vi "Enable.vi"(8 "output cluster":T1, 11 "Enum":T2=enum."Create Report") -> ()   [LabVIEW 2014]
uses:
  CMD UI enum.ctl
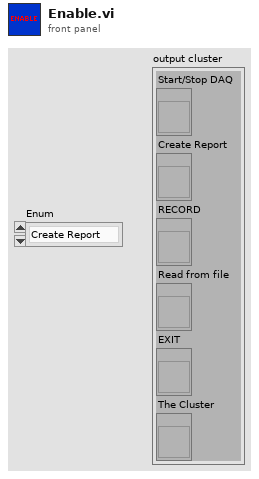
[diagram p1: front panel]
types:
  T1 = cluster{"Start/Stop DAQ":refnum<vi>, "Create Report":refnum<vi>, "RECORD":refnum<vi>, "Read from file":refnum<vi>, "EXIT":refnum<vi>, "The Cluster":refnum<vi>}
  T2 = typedef "CMD UI enum.ctl" = enum16{"Init all", "Update Patient Info", "Update Analyzed", "Create Report", "Analyze Data", "Start DAQ", "Start Read", "LOG Data", "Stop LOG Data", "Stop DAQ", "Stop Read", "EXIT"}
  T3 = enum8{"Enabled", "Disabled", "Disabled and Grayed Out"}
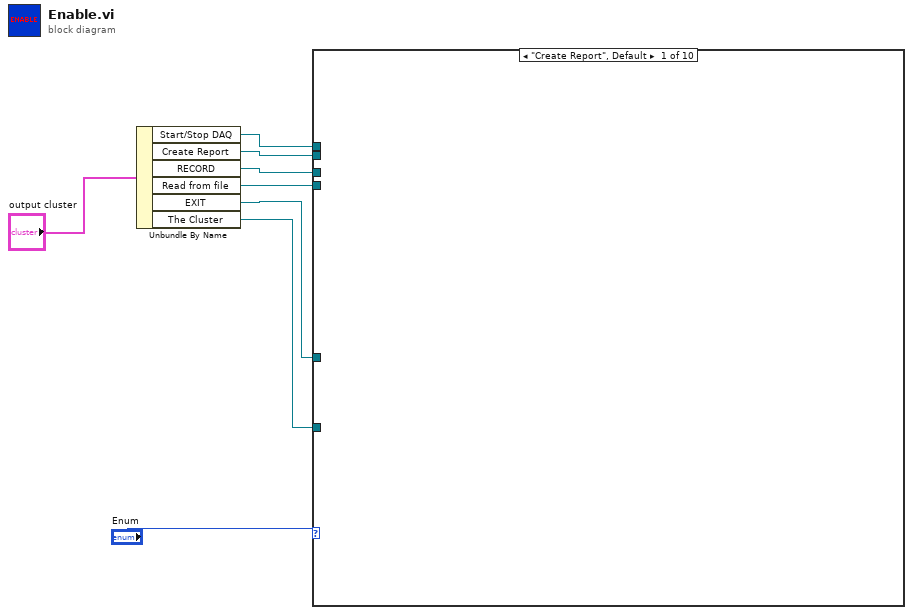
[diagram p0: block diagram]
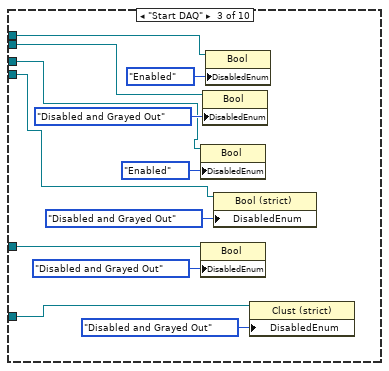
[diagram p3: hidden frame]
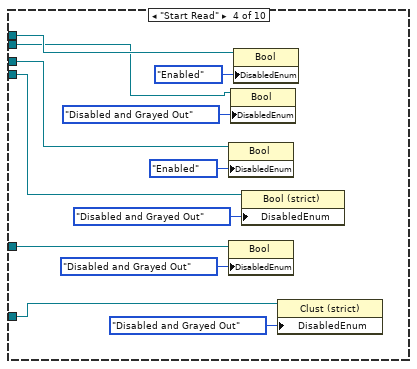
[diagram p4: hidden frame]
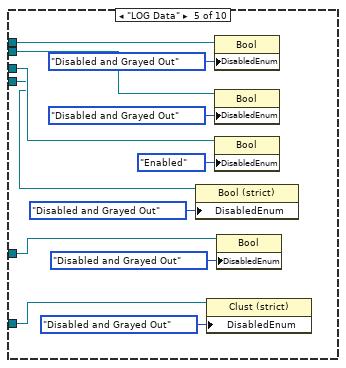
[diagram p5: hidden frame]
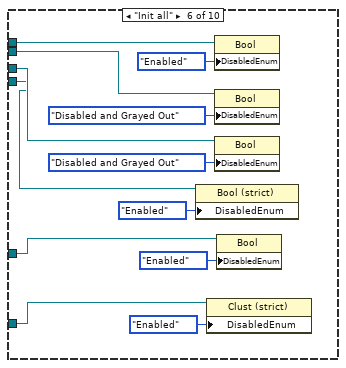
[diagram p6: hidden frame]
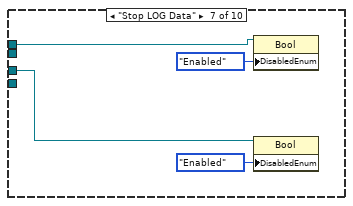
[diagram p7: hidden frame]
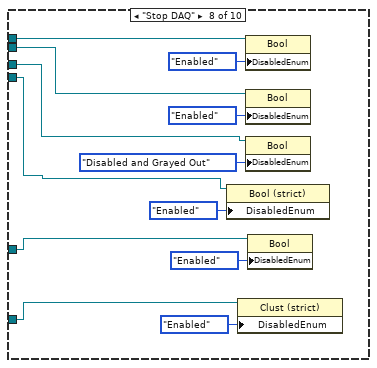
[diagram p8: hidden frame]
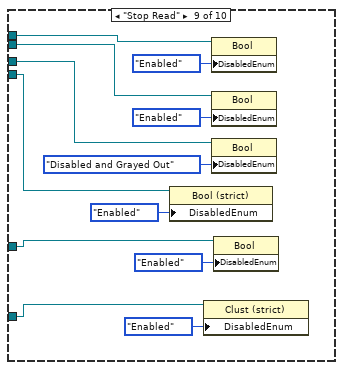
[diagram p9: hidden frame]
diagram:
  n1 = Unbundle By Name("output cluster") -> ("Start/Stop DAQ"=w7:refnum<vi>, "Create Report"=w6:refnum<vi>, "RECORD"=w5:refnum<vi>, "Read from file"=w3:refnum<vi>, "EXIT"=w2:refnum<vi>, "The Cluster"=w4:refnum<vi>)
  n2 = case shown="\"Create Report\", Default" "Enum" {
    tunnel: w7 -> [_ _ w15 w26 w44 w56 w58 w66 w78 _]
    tunnel: w6 -> [_ _ w14 w25 w43 w55 _ w65 w77 _]
    tunnel: w5 -> [_ _ w13 w24 w42 w54 w57 w64 w76 _]
    tunnel: w2 -> [_ _ w12 w22 w39 w51 _ w62 w74 _]
    tunnel: w4 -> [_ _ w10 w21 w40 w52 _ w61 w73 _]
    tunnel: w3 -> [_ _ w9 w23 w41 w53 _ w63 w75 _]
    frame "Create Report", Default {
    }
    frame "Analyze Data" {
    }
    frame "Start DAQ" {
      n3 = property on="Property Node" class="Bool"(reference=w13, "DisabledEnum"=T3."Enabled" ("Disabled")) -> ()  [unwired: 1 in, 2 out]
      n4 = property on="Property Node" class="Bool"(reference=w12, "DisabledEnum"=T3."Disabled and Grayed Out" ("Disabled")) -> ()  [unwired: 1 in, 2 out]
      n5 = property on="Property Node" class="Bool"(reference=w14, "DisabledEnum"=T3."Disabled and Grayed Out" ("Disabled")) -> ()  [unwired: 1 in, 2 out]
      n6 = property on="Property Node" class="Bool"(reference=w15, "DisabledEnum"=T3."Enabled" ("Disabled")) -> ()  [unwired: 1 in, 2 out]
      n7 = property on="Property Node" class="Bool (strict)"(reference=w9, "DisabledEnum"=T3."Disabled and Grayed Out" ("Disabled")) -> ()  [unwired: 1 in, 2 out]
      n8 = property on="Property Node" class="Clust (strict)"(reference=w10, "DisabledEnum"=T3."Disabled and Grayed Out" ("Disabled")) -> ()  [unwired: 1 in, 2 out]
    }
    frame "Start Read" {
      n9 = property on="Property Node" class="Bool"(reference=w24, "DisabledEnum"=T3."Enabled" ("Disabled")) -> ()  [unwired: 1 in, 2 out]
      n10 = property on="Property Node" class="Bool"(reference=w22, "DisabledEnum"=T3."Disabled and Grayed Out" ("Disabled")) -> ()  [unwired: 1 in, 2 out]
      n11 = property on="Property Node" class="Bool"(reference=w25, "DisabledEnum"=T3."Disabled and Grayed Out" ("Disabled")) -> ()  [unwired: 1 in, 2 out]
      n12 = property on="Property Node" class="Bool"(reference=w26, "DisabledEnum"=T3."Enabled" ("Disabled")) -> ()  [unwired: 1 in, 2 out]
      n13 = property on="Property Node" class="Bool (strict)"(reference=w23, "DisabledEnum"=T3."Disabled and Grayed Out" ("Disabled")) -> ()  [unwired: 1 in, 2 out]
      n14 = property on="Property Node" class="Clust (strict)"(reference=w21, "DisabledEnum"=T3."Disabled and Grayed Out" ("Disabled")) -> ()  [unwired: 1 in, 2 out]
    }
    frame "LOG Data" {
      n15 = property on="Property Node" class="Bool (strict)"(reference=w41, "DisabledEnum"=T3."Disabled and Grayed Out" ("Disabled")) -> ()  [unwired: 1 in, 2 out]
      n16 = property on="Property Node" class="Clust (strict)"(reference=w40, "DisabledEnum"=T3."Disabled and Grayed Out" ("Disabled")) -> ()  [unwired: 1 in, 2 out]
      n17 = property on="Property Node" class="Bool"(reference=w44, "DisabledEnum"=T3."Disabled and Grayed Out" ("Disabled")) -> ()  [unwired: 1 in, 2 out]
      n18 = property on="Property Node" class="Bool"(reference=w43, "DisabledEnum"=T3."Disabled and Grayed Out" ("Disabled")) -> ()  [unwired: 1 in, 2 out]
      n19 = property on="Property Node" class="Bool"(reference=w42, "DisabledEnum"=T3."Enabled" ("Disabled")) -> ()  [unwired: 1 in, 2 out]
      n20 = property on="Property Node" class="Bool"(reference=w39, "DisabledEnum"=T3."Disabled and Grayed Out" ("Disabled")) -> ()  [unwired: 1 in, 2 out]
    }
    frame "Init all" {
      n21 = property on="Property Node" class="Bool (strict)"(reference=w53, "DisabledEnum"=T3."Enabled" ("Disabled")) -> ()  [unwired: 1 in, 2 out]
      n22 = property on="Property Node" class="Clust (strict)"(reference=w52, "DisabledEnum"=T3."Enabled" ("Disabled")) -> ()  [unwired: 1 in, 2 out]
      n23 = property on="Property Node" class="Bool"(reference=w56, "DisabledEnum"=T3."Enabled" ("Disabled")) -> ()  [unwired: 1 in, 2 out]
      n24 = property on="Property Node" class="Bool"(reference=w55, "DisabledEnum"=T3."Disabled and Grayed Out" ("Disabled")) -> ()  [unwired: 1 in, 2 out]
      n25 = property on="Property Node" class="Bool"(reference=w54, "DisabledEnum"=T3."Disabled and Grayed Out" ("Disabled")) -> ()  [unwired: 1 in, 2 out]
      n26 = property on="Property Node" class="Bool"(reference=w51, "DisabledEnum"=T3."Enabled" ("Disabled")) -> ()  [unwired: 1 in, 2 out]
    }
    frame "Stop LOG Data" {
      n27 = property on="Property Node" class="Bool"(reference=w58, "DisabledEnum"=T3."Enabled" ("Disabled")) -> ()  [unwired: 1 in, 2 out]
      n28 = property on="Property Node" class="Bool"(reference=w57, "DisabledEnum"=T3."Enabled" ("Disabled")) -> ()  [unwired: 1 in, 2 out]
    }
    frame "Stop DAQ" {
      n29 = property on="Property Node" class="Bool (strict)"(reference=w63, "DisabledEnum"=T3."Enabled" ("Disabled")) -> ()  [unwired: 1 in, 2 out]
      n30 = property on="Property Node" class="Clust (strict)"(reference=w61, "DisabledEnum"=T3."Enabled" ("Disabled")) -> ()  [unwired: 1 in, 2 out]
      n31 = property on="Property Node" class="Bool"(reference=w66, "DisabledEnum"=T3."Enabled" ("Disabled")) -> ()  [unwired: 1 in, 2 out]
      n32 = property on="Property Node" class="Bool"(reference=w65, "DisabledEnum"=T3."Enabled" ("Disabled")) -> ()  [unwired: 1 in, 2 out]
      n33 = property on="Property Node" class="Bool"(reference=w64, "DisabledEnum"=T3."Disabled and Grayed Out" ("Disabled")) -> ()  [unwired: 1 in, 2 out]
      n34 = property on="Property Node" class="Bool"(reference=w62, "DisabledEnum"=T3."Enabled" ("Disabled")) -> ()  [unwired: 1 in, 2 out]
    }
    frame "Stop Read" {
      n35 = property on="Property Node" class="Bool (strict)"(reference=w75, "DisabledEnum"=T3."Enabled" ("Disabled")) -> ()  [unwired: 1 in, 2 out]
      n36 = property on="Property Node" class="Clust (strict)"(reference=w73, "DisabledEnum"=T3."Enabled" ("Disabled")) -> ()  [unwired: 1 in, 2 out]
      n37 = property on="Property Node" class="Bool"(reference=w78, "DisabledEnum"=T3."Enabled" ("Disabled")) -> ()  [unwired: 1 in, 2 out]
      n38 = property on="Property Node" class="Bool"(reference=w77, "DisabledEnum"=T3."Enabled" ("Disabled")) -> ()  [unwired: 1 in, 2 out]
      n39 = property on="Property Node" class="Bool"(reference=w76, "DisabledEnum"=T3."Disabled and Grayed Out" ("Disabled")) -> ()  [unwired: 1 in, 2 out]
      n40 = property on="Property Node" class="Bool"(reference=w74, "DisabledEnum"=T3."Enabled" ("Disabled")) -> ()  [unwired: 1 in, 2 out]
    }
    frame "EXIT" {
    }
  }
